vi "Stop Print.vi"(8 "error in (no error)":errorcluster, 11 "Feeder Actor.lvlib:Feeder.lvclass":refnum<class "Feeder.lvclass">) -> (0 "error out":errorcluster, 3 "Feeder Actor.lvlib:Feeder.lvclass 2":refnum<class "Feeder.lvclass">)   [LabVIEW 2018, in "Feeder Actor.lvlib" / "Feeder.lvclass"]
uses:
  Feeder.lvclass
  Feeder.lvclass/Feeder.ctl
  Mixer Messages/Change Mixer Msg/Set Mixer Msg.lvclass/Set Mixer Msg.ctl
  <vilib>/ActorFramework/Message Enqueuer/Message Enqueuer.lvclass/Message Enqueuer.ctl
  Screw Messages/Change Screw Msg/Set Screw Msg.lvclass/Set Screw Msg.ctl
  Solenoid Messages/Set Solonoid Msg/Set Solonoid Msg.lvclass/Set Solonoid Msg.ctl
  <vilib>/ActorFramework/Message Enqueuer/Enqueue.vi
  Mixer Messages/Change Mixer Msg/Set Mixer Msg.lvclass
  C:/Program Files/National Instruments/LabVIEW 2018/vi.lib/ActorFramework/Message/Message.lvclass
  Screw Messages/Change Screw Msg/Set Screw Msg.lvclass
  Solenoid Messages/Set Solonoid Msg/Set Solonoid Msg.lvclass
  <vilib>/ActorFramework/Message Priority Queue/Priority Enqueue.vi
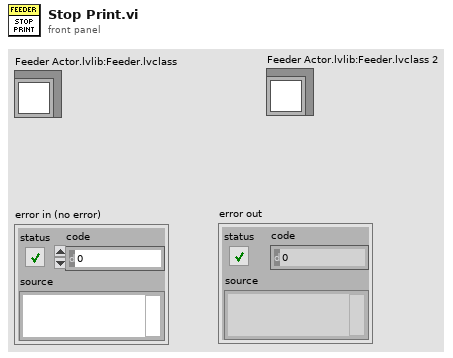
[diagram p1: front panel]
types:
  T1 = enum8{"Enabled", "Disabled", "Disabled and Grayed Out"}
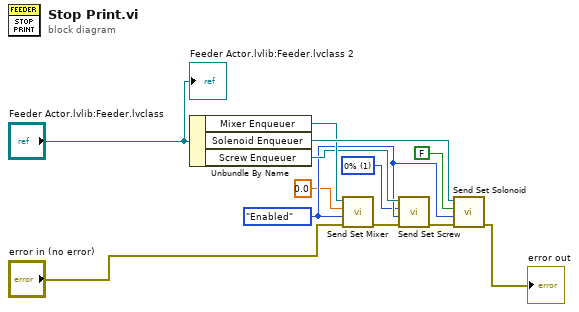
[diagram p0: block diagram]
diagram:
  w5 = u16 1 items=["0%"=1, "25%"=225, "50%"=450, "75%"=675, "100%"=900] ("Screw")
  w7 = T1."Enabled" ("Disabled")
  n1 = Unbundle By Name("Feeder Actor.lvlib:Feeder.lvclass") -> ("Mixer Enqueuer"=w9:refnum<class "Message Enqueuer.lvclass">, "Solenoid Enqueuer"=w11:refnum<class "Message Enqueuer.lvclass">, "Screw Enqueuer"=w8:refnum<class "Message Enqueuer.lvclass">)
  n2 = call "Send Set Mixer.vi"("error in (no error)"="error in (no error)", "Enabled?"=w7, "Mixer"=0.0, "Message Enqueuer"=w9) -> ("error out"=w4:errorcluster)  [unwired: 6 in, 1 out]
  n3 = call "Send Set Screw.vi"("error in (no error)"=w4, "Enabled?"=w7, "Screw"=w5, "Message Enqueuer"=w8) -> ("error out"=w3:errorcluster)  [unwired: 6 in, 1 out]
  n4 = call "Send Set Solonoid.vi"("error in (no error)"=w3, "Enabled?"=w7, "State"=FALSE, "Message Enqueuer in"=w11) -> ("error out"=→"error out":errorcluster)  [unwired: 6 in, 1 out]
  "Feeder Actor.lvlib:Feeder.lvclass 2" <- "Feeder Actor.lvlib:Feeder.lvclass"
